vi "Restart VISA Resource.vi"(8 "error in (no error)":errorcluster, 11 "VISA Refnum in":refnum<visa-resource-name>) -> (0 "error out":errorcluster, 3 "VISA resource name out":refnum<visa-resource-name>)   [LabVIEW 2020, in "ChromTech Next Gen Compensator Pump.lvlib" / "Instrument Manager.lvlib"]
uses:
  Instrument Manager.lvlib
  <instrlib>/RxnRover/ChromtechSeriesIIIDriver/ChromTech Series III Pump.lvlib
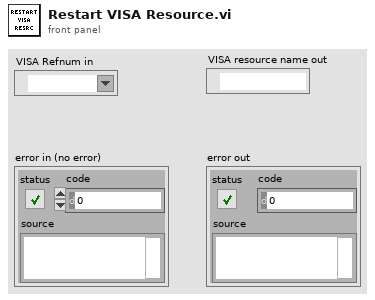
[diagram p1: front panel]
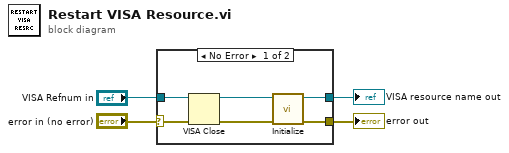
[diagram p0: block diagram]
diagram:
  n1 = case shown="No Error" "error in (no error)" {
    selector: "error in (no error)" -> [w6 w11]
    tunnel: "VISA Refnum in" -> [w9 w10]
    tunnel: [w7 w11] -> w3
    tunnel: [w5 w10] -> w1
    frame No Error {
      n2 = VISA Close(VISA resource name=w9, error in (no error)=w6) -> (error out=w8:errorcluster)
      n3 = call <instrlib>:"Initialize.vi"("error in (no error)"=w8, "VISA resource name"=w9) -> ("error out"=w7:errorcluster, "VISA resource name out"=w5:refnum<visa-resource-name>)  [unwired: 8 in]
    }
    frame Error {
    }
  }
  "error out" <- w3
  "VISA resource name out" <- w1
